vi "Initialize.vi"(8 "error in (no error)":errorcluster, 11 "Object ref in":T1) -> (0 "error out":errorcluster, 3 "Object ref out":T1)   [LabVIEW 2013, in "MaterialCharacterization.lvlib" / "MC-Main.lvclass"]
uses:
  MC-Main.lvclass
  Object-reference.ctl
  Application-status.ctl
  UI/Control-names.ctl
  MC-Main.lvclass/MC-Main.ctl
  Read UI.vi
  UI/MC-UI.lvclass
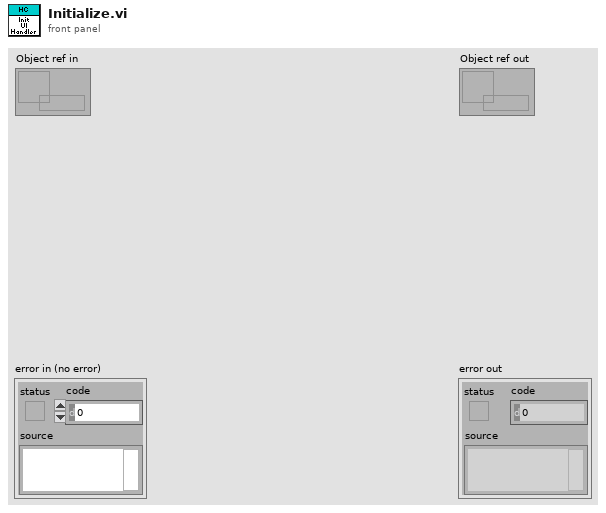
[diagram p1: front panel]
types:
  T1 = typedef "MaterialCharacterization.lvlib/MC-Main.lvclass/Object-reference.ctl" = refnum<data-value>
  T2 = typedef "MaterialCharacterization.lvlib/MC-Main.lvclass/Application-status.ctl" = enum16{"Idle", "Initialized", "Configured", "Activated", "Started", "Paused", "Stopped", "Reset", "Error", "Exited"}
  T3 = typedef "MaterialCharacterization.lvlib/MC-UI.lvclass/Control-names.ctl" = enum16{"Help", "Status", "Load configuration", "Save configuration", "Activate", "Start", "Stop", "Options"}
  T4 = typedef "MaterialCharacterization.lvlib/MC-UI.lvclass/Panes-reference.ctl" = refnum<data-value>
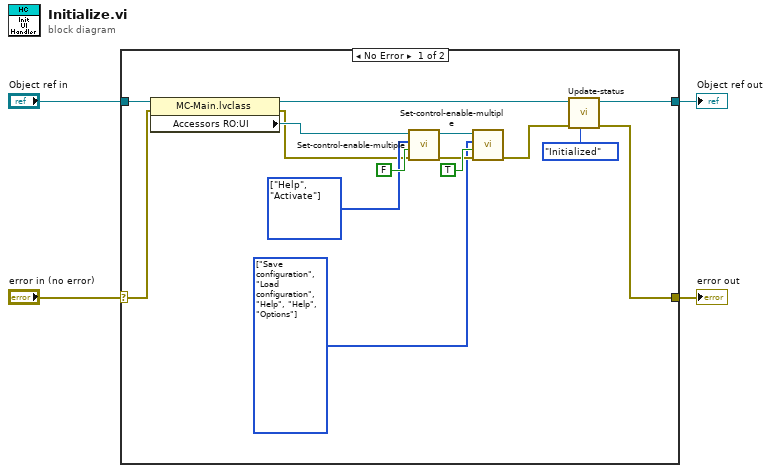
[diagram p0: block diagram]
diagram:
  n1 = case shown="No Error" "error in (no error)" {
    selector: "error in (no error)" -> [w14 w21]
    tunnel: [w18 w21] -> w3
    tunnel: [w17 w20] -> w1
    tunnel: "Object ref in" -> [w15 w20]
    frame No Error {
      w8 = T3[] [enum."Save configuration", enum."Load configuration", enum."Help", enum."Help", enum."Options"] items=["Help", "Status", "Load configuration", "Save configuration", "Activate", "Start", "Stop", "Options"] ("Control names")
      w9 = T3[] [enum."Help", enum."Activate"] items=["Help", "Status", "Load configuration", "Save configuration", "Activate", "Start", "Stop", "Options"] ("Control names")
      n2 = property class="MC-Main.lvclass"(reference=w15, error in=w14) -> (reference out=w16:T1, error out=w6:errorcluster, "Accessors RO:UI"=w7:T4)
      n3 = call "Set-control-enable-multiple.vi"("error in (no error)"=w6, "Enable?"=FALSE, "Control names"=w9, "Panes in"=w7) -> ("error out"=w10:errorcluster, "Panes out"=w13:T4)  [unwired: 6 in]
      n4 = call "Set-control-enable-multiple.vi"("error in (no error)"=w10, "Enable?"=TRUE, "Control names"=w8, "Panes in"=w13) -> ("error out"=w5:errorcluster)  [unwired: 6 in, 1 out]
      n5 = call "Update-status.vi"("Status"=Application-status."Initialized", "error in (no error)"=w5, "Object ref in"=w16) -> ("error out"=w18:errorcluster, "Object ref out"=w17:T1)  [unwired: 7 in]
    }
    frame Error {
    }
  }
  "error out" <- w3
  "Object ref out" <- w1
